vi "test Connect.vi"(8 "error in (no error)":errorcluster, 11 "TestCase in":refnum<class "Test TCP Stream Initiator Connect.lvclass">) -> (0 "error out":errorcluster, 3 "TestCase out":refnum<class "Test TCP Stream Initiator Connect.lvclass">)   [LabVIEW 2020, in "Test TCP Stream Initiator Connect.lvclass"]
uses:
  Test TCP Stream Initiator Connect.lvclass
  <vilib>/addons/_JKI Toolkits/VI Tester/TestCase.llb/TestCase.lvclass
  Source/Protocols/TCP Strategy/TCP Stream Initiator/TCP Stream Initiator.lvclass
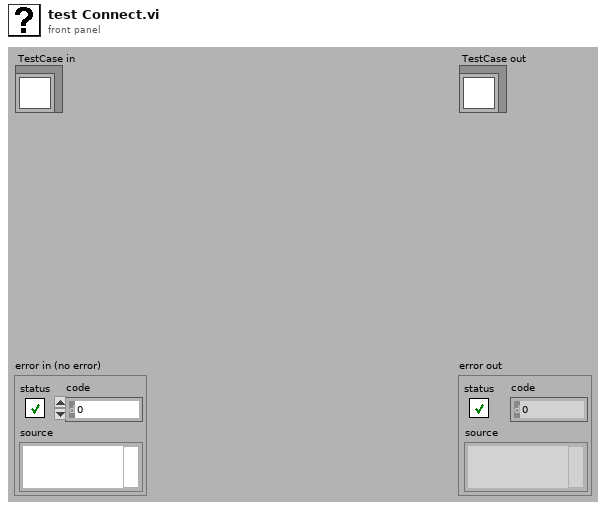
[diagram p1: front panel]
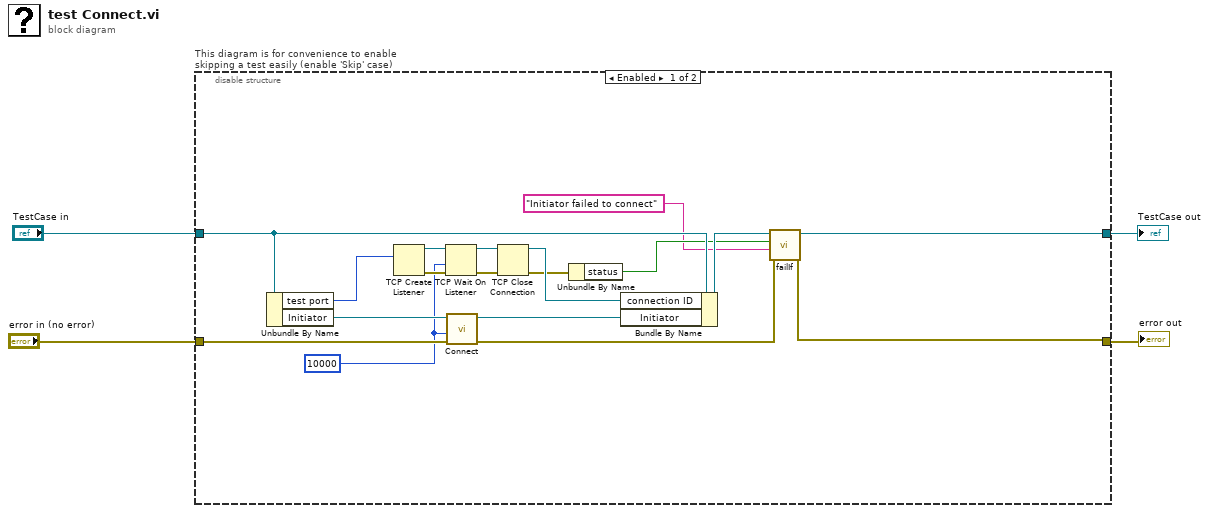
[diagram p0: block diagram]
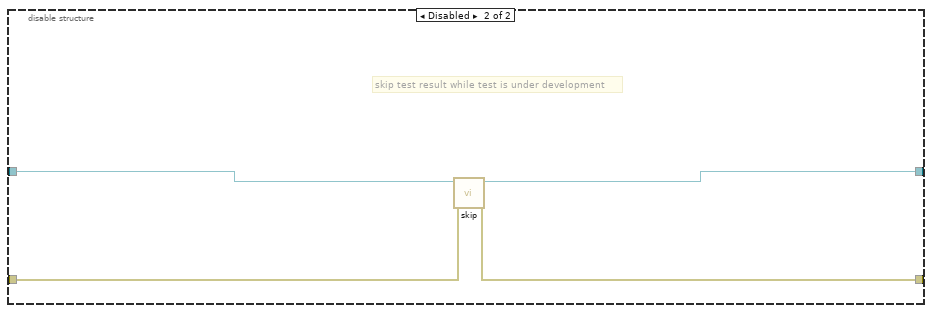
[diagram p2: hidden frame]
diagram:
  n1 = disable-structure "This diagram is for convenience to enable skipping a test easily (enable 'Skip' case)" shown="Enabled" {
    disable-tunnel: "TestCase in" -> [w17 w26]
    disable-tunnel: [w22 w24] -> w1
    disable-tunnel: [w21 w25] -> w3
    disable-tunnel: "error in (no error)" -> [w20 w23]
    frame Enabled {
      w5 = 10000 ("timeout")
      n2 = Unbundle By Name(w17) -> ("test port"=w10:u16, "Initiator"=w18:refnum<class "TCP Stream Initiator.lvclass">)
      n3 = TCP Create Listener(10:w10) -> (0:w14:errorcluster, 3:w13:refnum<k5>)  [unwired: 4 in, 1 out]
      n4 = TCP Wait On Listener(8:w14, 9:w5, 11:w13) -> (0:w12:errorcluster, 3:w11:refnum<k5>)  [unwired: 1 in, 3 out]
      n5 = call-dynamic "Connect.vi"("error in (no error)"=w20, "timeout"=w5, "TCP Stream Initiator in"=w18) -> ("error out"=w19:errorcluster, "TCP Stream Initiator out"=w15:refnum<class "TCP Stream Initiator.lvclass">)  [unwired: 7 in]
      n6 = TCP Close Connection(connection ID=w11, error in (no error)=w12) -> (connection ID out=w9:refnum<k5>, error out=w8:errorcluster)  [unwired: 1 in]
      n7 = Unbundle By Name(w8) -> ("status"=w7:bool)
      n8 = Bundle By Name(cluster=w17, "connection ID"=w9, "Initiator"=w15) -> (w16:refnum<class "Test TCP Stream Initiator Connect.lvclass">)
      n9 = call-dynamic "failIf.vi"("error in (no error)"=w19, "message (\"\")"="Initiator failed to connect" ("message (\"\")"), "fail"=w7, "TestCase in"=w16) -> ("error out"=w21:errorcluster, "TestCase out"=w22:refnum<class "Test TCP Stream Initiator Connect.lvclass">)  [unwired: 6 in]
    }
    frame Disabled {
      # "skip test result while test is under development"
      n10 = call <vilib>:"skip.vi"("error in (no error)"=w23, "TestCase in"=w26) -> ("error out"=w25:errorcluster, "TestCase out"=w24:refnum<class "Test TCP Stream Initiator Connect.lvclass">)  [unwired: 8 in]
    }
  }
  "error out" <- w3
  "TestCase out" <- w1
